vi "Get Pressure Offsets.vi"(8 "Error In":errorcluster, 11 "Path":path) -> (0 "Error Out":errorcluster, 3 "Pressure Offsets":dbl[](array[numeric]))   [LabVIEW 2013]
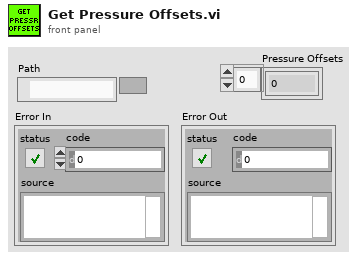
[diagram p1: front panel]
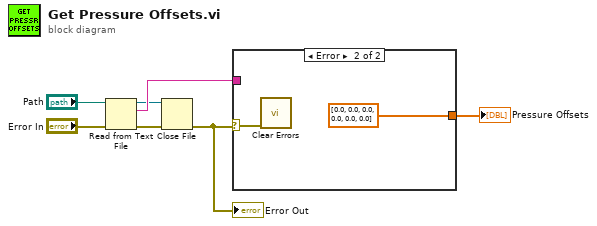
[diagram p0: block diagram]
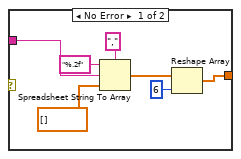
[diagram p2: hidden frame]
diagram:
  n1 = Read from Text File(file (use dialog)="Path", error in="Error In") -> (refnum out=w6:refnum<file>, text=w7:string, error out=w5:errorcluster)  [unwired: 2 in, 1 out]
  n2 = Close File(refnum=w6, error in=w5) -> (error out=w3:errorcluster)  [unwired: 1 out]
  "Error Out" <- w3
  n3 = case shown="Error" w3 {
    selector: w3 -> [_ w16]
    tunnel: w7 -> [w12 _]
    tunnel: [w8 dbl[] [0.0, 0.0, 0.0, 0.0, 0.0, 0.0]] -> w1
    frame No Error {
      n4 = Spreadsheet String To Array(delimiter (Tab)=",", format string="%.2f", spreadsheet string=w12, array type (2D Dbl)=dbl[] []) -> (array=w10:dbl[])
      n5 = Reshape Array(w10, 6 ("dimension size")) -> (w8:dbl[])
    }
    frame Error {
      n6 = call <vilib>:"Clear Errors.vi"("error in (no error)"=w16) -> ()  [unwired: 6 in, 1 out]
    }
  }
  "Pressure Offsets" <- w1
